vi "03-Vending1.vi"() -> ()   [LabVIEW 2017]
uses:
  Support/03-Typedef.ctl
panel:
  in  "100 Yen":bool
  in  "Change":bool
  out "Current Value":i32
  in  "Vend":bool
  in  "stop":bool
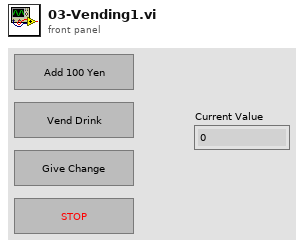
[diagram p1: front panel]
types:
  T1 = typedef "03-Typedef.ctl" = enum16{"Init", "Vend", "Change", "Add Money", "Idle", "Exit"}
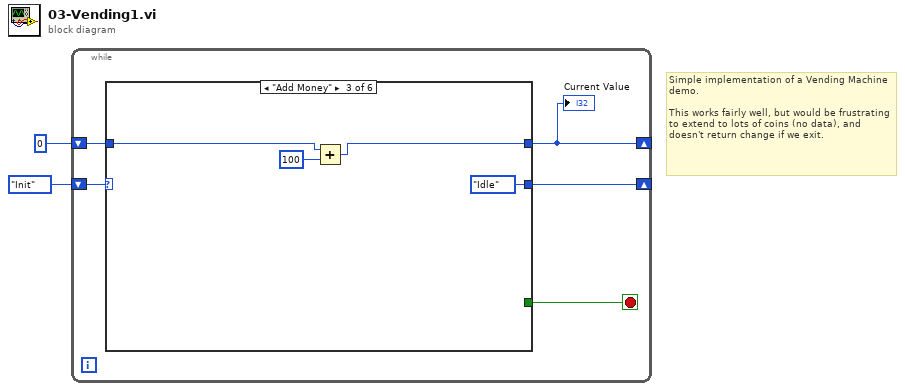
[diagram p0: block diagram]
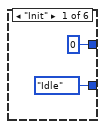
[diagram p2: hidden frame]
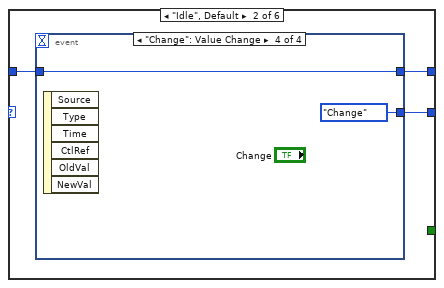
[diagram p3: hidden frame]
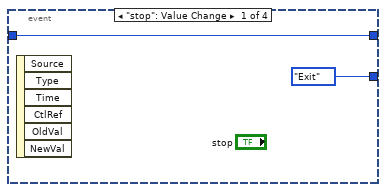
[diagram p4: hidden frame]
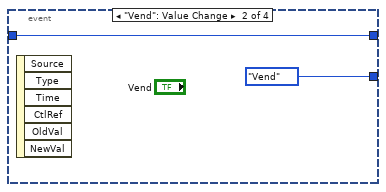
[diagram p5: hidden frame]
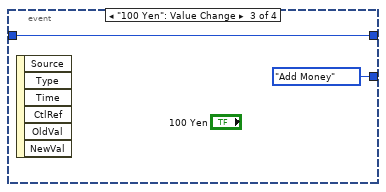
[diagram p6: hidden frame]
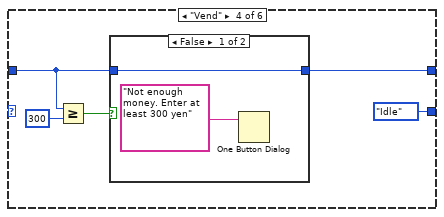
[diagram p7: hidden frame]
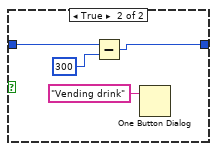
[diagram p8: hidden frame]
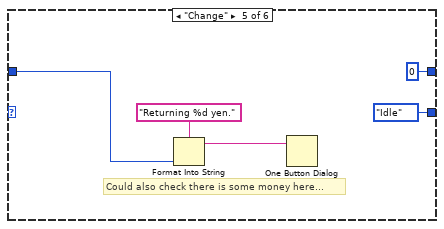
[diagram p9: hidden frame]
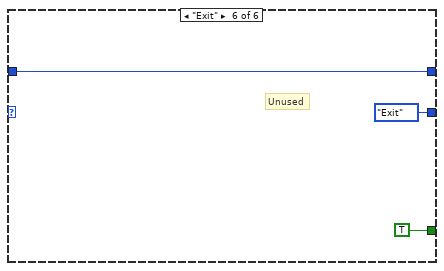
[diagram p10: hidden frame]
diagram:
  # "Simple implementation of a Vending Machine demo.\n\nThis works fairly well, but would be frustrating to extend to lots of coins (no data), and doesn't return change if we exit."
  n1 = while {
    shift-right: [w5] -> _
    shift-left: 03-Typedef."Init" ("Enum") -> [w7]
    shift-right: [w3] -> _
    shift-left: 0 -> [w4]
    stop <- w6 stop-if-true
    n2 = case shown="\"Add Money\"" w7 {
      tunnel: [_ _ _ _ _ TRUE] -> w6
      tunnel: [03-Typedef."Idle" ("Enum") w12 03-Typedef."Idle" ("Enum") 03-Typedef."Idle" ("Enum") 03-Typedef."Idle" ("Enum") 03-Typedef."Exit" ("Enum")] -> w5
      tunnel: w4 -> [_ w11 w24 w26 w37 w41]
      tunnel: [0 w10 w23 w25 0 w41] -> w3
      frame "Init" {
      }
      frame "Idle", Default {
        n3 = event shown="[3] \"Change\": Value Change" {
          selector: _ -> [_ _ _ _]
          dyn-events: _ -> [_ _ _ _]
          timeout: _ -> [_ _ _ _]
          tunnel: [03-Typedef."Exit" ("t") 03-Typedef."Vend" ("Enum") 03-Typedef."Add Money" ("Enum") 03-Typedef."Change" ("Enum")] -> w12
          tunnel: w11 -> [w13 w15 w17 w20]
          tunnel: [w13 w15 w17 w20] -> w10
          event "stop": Value Change {
            n4 = event-data() -> ()  [unwired: 1 in, 6 out]
          }
          event "Vend": Value Change {
            n5 = event-data() -> ()  [unwired: 1 in, 6 out]
          }
          event "100 Yen": Value Change {
            n6 = event-data() -> ()  [unwired: 1 in, 6 out]
          }
          event "Change": Value Change {
            n7 = event-data() -> ()  [unwired: 1 in, 6 out]
          }
        }
      }
      frame "Add Money" {
        n8 = Add(x=w24, y=100) -> (x+y=w23:i32)
      }
      frame "Vend" {
        n9 = Greater Or Equal?(x=w26, y=300) -> (x >= y?=w27:bool)
        n10 = case shown="False" w27 {
          tunnel: w26 -> [w30 w34]
          tunnel: [w30 w32] -> w25
          frame False {
            n11 = One Button Dialog(message="Not enough money. Enter at least 300 yen") -> ()  [unwired: 1 in, 1 out]
          }
          frame True {
            n12 = Subtract(x=w34, y=300) -> (x-y=w32:i32)
            n13 = One Button Dialog(message="Vending drink") -> ()  [unwired: 1 in, 1 out]
          }
        }
      }
      frame "Change" {
        # "Could also check there is some money here..."
        n14 = Format Into String(format string="Returning %d yen.", w37) -> (resulting string=w39:string)  [unwired: 2 in, 1 out]
        n15 = One Button Dialog(message=w39) -> ()  [unwired: 1 in, 1 out]
      }
      frame "Exit" {
        # "Unused"
      }
    }
    "Current Value" <- w3
  }
